vi "loadItems.vi"(8 "error in (no error)":errorcluster) -> (0 "error out":errorcluster, 3 "Array":T1[](array[typedef]))   [LabVIEW 2021]
uses:
  Item.ctl
  <vilib>/Utility/config.llb/Read Key (String).vi
  <vilib>/Utility/config.llb/Read Key (Double).vi
  <vilib>/Utility/config.llb/NI_LVConfig.lvlib
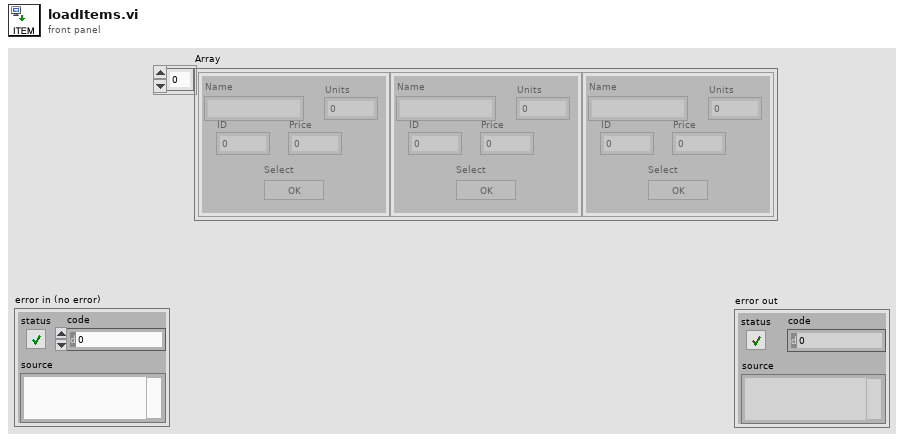
[diagram p1: front panel]
types:
  T1 = typedef "Item.ctl" = cluster{"Name":string, "ID":dbl, "Price":dbl, "Select":bool, "Units":dbl}
  T2 = typedef "NI_LVConfig.lvlib/Config Data RefNum.ctl" = refnum<k1>
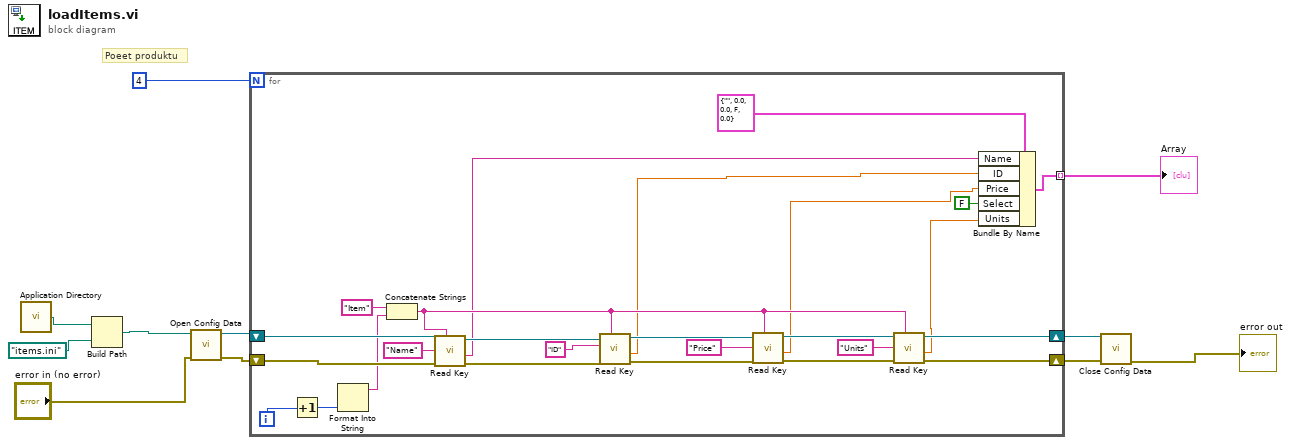
[diagram p0: block diagram]
diagram:
  # "Poeet produktu"
  n1 = call <vilib>:"Application Directory.vi"() -> ("Application Directory"=w3:path)
  n2 = Build Path(base path=w3, name or relative path=path "items.ini") -> (appended path=w1:path)
  n3 = call <vilib>:"Open Config Data.vi"("error in (no error)"="error in (no error)", "configuration file path"=w1) -> ("error out"=w11:errorcluster, "refnum"=w7:T2)  [unwired: 7 in, 1 out]
  n4 = for {
    N: 4 -> [_]
    shift-right: [w33] -> w10
    shift-left: w11 -> [w37]
    tunnel: [w21] -> w4 mode=indexing
    shift-right: [w27] -> w6
    shift-left: w7 -> [w31]
    i -> [w16]
    n5 = Increment(x=w16) -> (x+1=w15:i32)
    n6 = Format Into String(w15) -> (resulting string=w26:string)  [unwired: 3 in, 1 out]
    n7 = Concatenate Strings("Item" ("section"), w26) -> (w24:string)
    n8 = call-poly <vilib>:"Read Key.vi"("section"=w24, "error in (no error)"=w37, "key"="Name", "refnum"=w31) -> ("error out"=w36:errorcluster, "value"=w22:string, "refnum out"=w30:T2)  [unwired: 4 in, 1 out]
    n9 = call-poly <vilib>:"Read Key.vi"("section"=w24, "error in (no error)"=w36, "key"="ID", "refnum"=w30) -> ("error out"=w35:errorcluster, "value"=w14:dbl, "refnum out"=w29:T2)  [unwired: 4 in, 1 out]
    n10 = call-poly <vilib>:"Read Key.vi"("section"=w24, "error in (no error)"=w35, "key"="Price", "refnum"=w29) -> ("error out"=w34:errorcluster, "value"=w12:dbl, "refnum out"=w28:T2)  [unwired: 4 in, 1 out]
    n11 = call-poly <vilib>:"Read Key.vi"("section"=w24, "error in (no error)"=w34, "key"="Units", "refnum"=w28) -> ("error out"=w33:errorcluster, "value"=w13:dbl, "refnum out"=w27:T2)  [unwired: 4 in, 1 out]
    n12 = Bundle By Name(cluster=T1 {"Name"="", "ID"=0.0, "Price"=0.0, "Select"=FALSE, "Units"=0.0} ("Item"), "Name"=w22, "ID"=w14, "Price"=w12, "Select"=FALSE, "Units"=w13) -> (w21:T1)
  }
  "Array" <- w4
  n13 = call <vilib>:"Close Config Data.vi"("error in (no error)"=w10, "refnum"=w6) -> ("error out"=→"error out":errorcluster)  [unwired: 8 in, 1 out]
